vi "Destroy User Events.vi"(11 "UI Template in":refnum<class "Linear Encoder.lvclass">) -> (3 "UI Template out":refnum<class "Linear Encoder.lvclass">)   [LabVIEW 2020, in "Linear Encoder.lvlib" / "Linear Encoder.lvclass"]
uses:
  Linear Encoder.lvclass
  Linear Encoder.lvclass/Linear Encoder.ctl
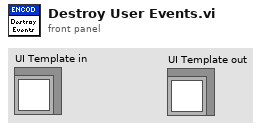
[diagram p1: front panel]
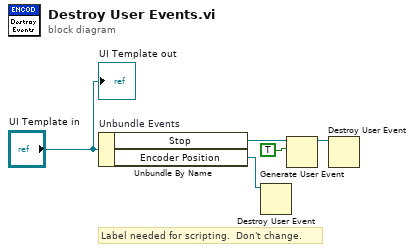
[diagram p0: block diagram]
diagram:
  # "Label needed for scripting.  Don't change."
  n1 = Unbundle By Name "Unbundle Events"("UI Template in") -> ("Stop"=w3:refnum<user-event>, "Encoder Position"=w1:refnum<user-event>)
  n2 = Destroy User Event(user event=w1) -> ()  [unwired: 1 in, 1 out]
  n3 = Generate User Event(user event=w3, event data cluster=TRUE ("event data")) -> (user event out=w4:refnum<user-event>)  [unwired: 2 in, 1 out]
  n4 = Destroy User Event(user event=w4) -> ()  [unwired: 1 in, 1 out]
  "UI Template out" <- "UI Template in"
